vi "test_Add Single Ch. Comparison.vi"(8 "error in (no error)":errorcluster, 11 "TestCase in":refnum<class "Instrument Addon Scripting API Channels Unit Tests.lvclass">) -> (0 "error out":errorcluster, 3 "TestCase out":refnum<class "Instrument Addon Scripting API Channels Unit Tests.lvclass">)   [LabVIEW 2018, in "Instrument Addon Scripting API Channels Unit Tests.lvclass"]
uses:
  Instrument Addon Scripting API Channels Unit Tests.lvclass
  APIs/Scripting API/TypeDefs/Single Channel Comparison Settings.ctl
  Addon/Addon Shared/Types/Protocol Data Type.ctl
  Addon/Addon Shared/Types/Data Channel Type.ctl
  Instrument Addon Scripting API Channels Unit Tests.lvclass/Instrument Addon Scripting API Channels Unit Tests.ctl
  Addon/Addon Shared/SubVIs/Constants.vi
  <vilib>/NI/NI VeriStand Advanced SysDef API/_SubVIs/SysDef.Search.GUID.vi
  <vilib>/NI/NI VeriStand Advanced SysDef API/_SubVIs/SysDef.Search.GUIDs.vi
  APIs/Scripting API/Channels/Create Data Channel - Single Channel - Comparison.vi
  <vilib>/NI Veristand/Custom Device API/Get Item Property (U16).vi
  <vilib>/NI Veristand/Custom Device API/Get Item Property (String).vi
  <vilib>/addons/_JKI Toolkits/VI Tester/TestCase.llb/TestCase.lvclass
  Instrument Addon Scripting API Test Assets/Instrument Addon Scripting API Test Assets.lvclass
  <vilib>/NI/NI VeriStand Advanced SysDef API/SysDef API/Advanced System Definition.lvlib
  Addon/Addon Shared/Instrument Addon Shared.lvlib
  <vilib>/NI Veristand/Custom Device API/Custom Device API.lvlib
  APIs/Scripting API/Instrument Addon Scripting API.lvlib
  C:/Program Files (x86)/National Instruments/LabVIEW 2018/vi.lib/addons/_JKI Toolkits/VI Tester/TestCase.llb/TestCase.lvclass
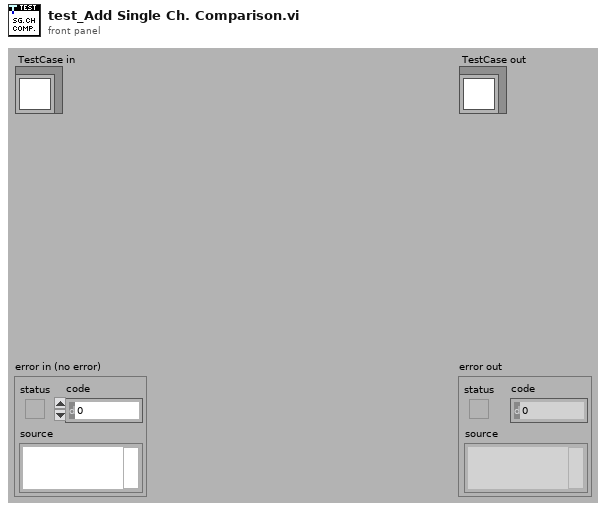
[diagram p1: front panel]
types:
  T1 = typedef "Instrument Addon Scripting API.lvlib/Single Channel Comparison Settings.ctl" = cluster{"Expected String(case sensitive)":string, "Default Value":dbl, "Units":string}
  T2 = typedef "Instrument Addon Shared.lvlib/Data Channel Type.ctl" = enum16{"Format", "Comparison", "Type Cast", "Enumerated List"}
  T3 = typedef "Instrument Addon Shared.lvlib/Protocol Data Type.ctl" = enum16{"Single Channel", "Array"}
  T4 = typedef "Custom Device API.lvlib/Custom Device Item Ref.ctl" = u64
  T5 = typedef "Custom Device API.lvlib/Custom Device Channel.ctl" = cluster{"Type":T6, "Units":string, "Default Value":dbl, "Faultable":bool, "Scalable":bool}
  T6 = typedef "Custom Device API.lvlib/Custom Device Channel Type.ctl" = enum16{"Input", "Output"}
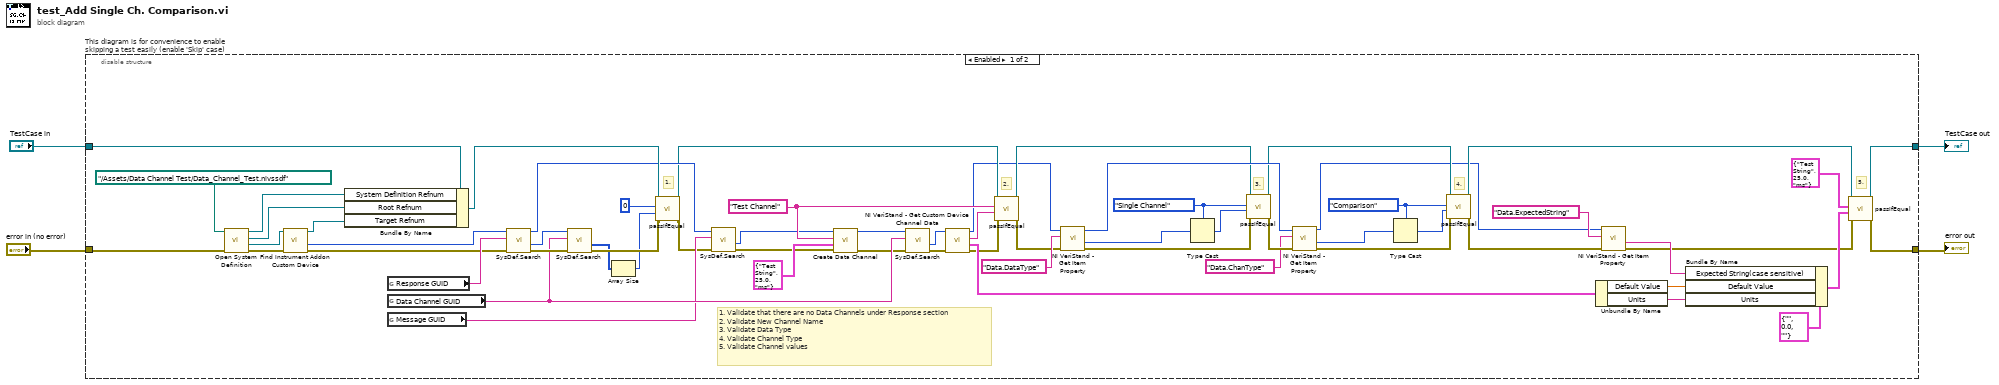
[diagram p0: block diagram]
diagram:
  n1 = disable-structure "This diagram is for convenience to enable skipping a test easily (enable 'Skip' case)" shown="Enabled" {
    disable-tunnel: "TestCase in" -> [w35 w71]
    disable-tunnel: [w67 w69] -> w1
    disable-tunnel: [w66 w70] -> w3
    disable-tunnel: "error in (no error)" -> [w63 w68]
    frame Enabled {
      w15 = Data_Channel_Type."Comparison" ("Channel Type")
      w20 = Protocol_Data_Type."Single Channel" ("Data Type")
      w46 = "Test Channel" ("Name")
      # "1. Validate that there are no Data Channels under Response section\n2. Validate New Channel Name\n3. Validate Data Type\n4. Validate Channel Type\n5. Validate Channel values"
      # "4."
      # "3."
      # "5."
      # "2."
      # "1."
      n2 = call "Open System Definition.vi"("error in (no error)"=w63, "System Definition File"=path "../Assets/Data Channel Test/Data_Channel_Test.nivssdf") -> ("error out"=w65:errorcluster, "Target Refnum"=w33:refnum<k24>, "Root Refnum"=w37:refnum<k24>, "System Definition Refnum"=w38:refnum<k24>)  [unwired: 6 in]
      n3 = call "Find Instrument Addon Custom Device.vi"("error in"=w65, "target in"=w33) -> ("error out"=w32:errorcluster, "NodeID"=w62:u64, "target out"=w36:refnum<k24>)  [unwired: 7 in]
      n4 = Bundle By Name(cluster=w35, "System Definition Refnum"=w38, "Root Refnum"=w37, "Target Refnum"=w36) -> (w34:refnum<class "Instrument Addon Scripting API Channels Unit Tests.lvclass">)
      n5 = global read "Constants.vi" "Response GUID"() -> (w61:string)
      n6 = global read "Constants.vi" "Data Channel GUID"() -> (w58:string)
      n7 = global read "Constants.vi" "Message GUID"() -> (w31:string)
      n8 = call-poly <vilib>:"SysDef.Search.vi"("error in (no error)"=w32, "GUID"=w61, "nodeID"=w62) -> ("error out"=w59:errorcluster, "Value out"=w60:u64, "nodeID out"=w28:u64)  [unwired: 5 in, 1 out]
      n9 = call-poly <vilib>:"SysDef.Search.vi"("error in (no error)"=w59, "GUID"=w58, "nodeID"=w60) -> ("error out"=w50:errorcluster, "Values Out"=w49:u64[])  [unwired: 5 in, 2 out]
      n10 = Array Size(array=w49) -> (size(s)=w48:i32)
      n11 = call-dynamic "passIfEqual.vi"("error in (no error)"=w50, "y"=w48, "x"=0 ("size(s)"), "TestCase in"=w34) -> ("error out"=w30:errorcluster, "TestCase out"=w25:refnum<class "Instrument Addon Scripting API Channels Unit Tests.lvclass">)  [unwired: 6 in]
      n12 = call-poly <vilib>:"SysDef.Search.vi"("error in (no error)"=w30, "GUID"=w31, "nodeID"=w28) -> ("error out"=w29:errorcluster, "Value out"=w27:u64)  [unwired: 5 in, 2 out]
      n13 = call-poly "Create Data Channel.vi"("Error In"=w29, "Settings"=T1 {"Expected String(case sensitive)"="Test String", "Default Value"=25.0, "Units"="ms"}, "Name"=w46, "Message Refnum In"=w27) -> ("Error Out"=w44:errorcluster, "Message Refnum Out"=w45:T4)  [unwired: 5 in, 1 out]
      n14 = call-poly <vilib>:"SysDef.Search.vi"("error in (no error)"=w44, "GUID"=w58, "nodeID"=w45) -> ("error out"=w57:errorcluster, "Value out"=w43:u64)  [unwired: 5 in, 2 out]
      n15 = call <vilib>:"NI VeriStand - Get Custom Device Channel Data.vi"("error in (no error)"=w57, "Channel Ref in"=w43) -> ("error out"=w26:errorcluster, "Channel"=w56:T5, "Channel Name"=w52:string, "Channel Ref out"=w9:T4)  [unwired: 4 in, 2 out]
      n16 = call-dynamic "passIfEqual.vi"("error in (no error)"=w26, "y"=w52, "x"=w46, "TestCase in"=w25) -> ("error out"=w11:errorcluster, "TestCase out"=w10:refnum<class "Instrument Addon Scripting API Channels Unit Tests.lvclass">)  [unwired: 6 in]
      n17 = call-poly <vilib>:"NI VeriStand - Get Item Property.vi"("error in (no error)"=w11, "Property Name"="Data.DataType", "Item Ref in"=w9) -> ("error out"=w23:errorcluster, "Value"=w22:u16, "Item Ref out"=w14:T4)  [unwired: 5 in, 1 out]
      n18 = Type Cast(type=w20, x=w22) -> (*(type *) &x=w21:T3)
      n19 = call-dynamic "passIfEqual.vi"("error in (no error)"=w23, "y"=w21, "x"=w20, "TestCase in"=w10) -> ("error out"=w19:errorcluster, "TestCase out"=w12:refnum<class "Instrument Addon Scripting API Channels Unit Tests.lvclass">)  [unwired: 6 in]
      n20 = call-poly <vilib>:"NI VeriStand - Get Item Property.vi"("error in (no error)"=w19, "Property Name"="Data.ChanType", "Item Ref in"=w14) -> ("error out"=w18:errorcluster, "Value"=w17:u16, "Item Ref out"=w5:T4)  [unwired: 5 in, 1 out]
      n21 = Type Cast(type=w15, x=w17) -> (*(type *) &x=w16:T2)
      n22 = call-dynamic "passIfEqual.vi"("error in (no error)"=w18, "y"=w16, "x"=w15, "TestCase in"=w12) -> ("error out"=w8:errorcluster, "TestCase out"=w7:refnum<class "Instrument Addon Scripting API Channels Unit Tests.lvclass">)  [unwired: 6 in]
      n23 = Unbundle By Name(w56) -> ("Default Value"=w55:dbl, "Units"=w54:string)
      n24 = call-poly <vilib>:"NI VeriStand - Get Item Property.vi"("error in (no error)"=w8, "Property Name"="Data.ExpectedString", "Item Ref in"=w5) -> ("error out"=w6:errorcluster, "Value"=w40:string)  [unwired: 5 in, 2 out]
      n25 = Bundle By Name(cluster=T1 {"Expected String(case sensitive)"="", "Default Value"=0.0, "Units"=""} ("Settings"), "Expected String(case sensitive)"=w40, "Default Value"=w55, "Units"=w54) -> (w51:T1)
      n26 = call-dynamic "passIfEqual.vi"("error in (no error)"=w6, "y"=w51, "x"=T1 {"Expected String(case sensitive)"="Test String", "Default Value"=25.0, "Units"="ms"} ("Settings"), "TestCase in"=w7) -> ("error out"=w66:errorcluster, "TestCase out"=w67:refnum<class "Instrument Addon Scripting API Channels Unit Tests.lvclass">)  [unwired: 6 in]
    }
    frame Disabled {
      # "skip test result while test is under development"
      n27 = call <vilib>:"skip.vi"("error in (no error)"=w68, "TestCase in"=w71) -> ("error out"=w70:errorcluster, "TestCase out"=w69:refnum<class "Instrument Addon Scripting API Channels Unit Tests.lvclass">)  [unwired: 8 in]
    }
  }
  "error out" <- w3
  "TestCase out" <- w1
